vi "Generate Dep Links.vi"(8 "error in":errorcluster, 9 "Dependency Names":string[](array[string]), 10 "Name":string, 11 "Create Unowned Container?":bool) -> (0 "error out":errorcluster, 3 "DGML Link Strings":string[](array[string]))   [LabVIEW 2018, in "DGML creation.lvlib"]
uses:
  DGML creation.lvlib
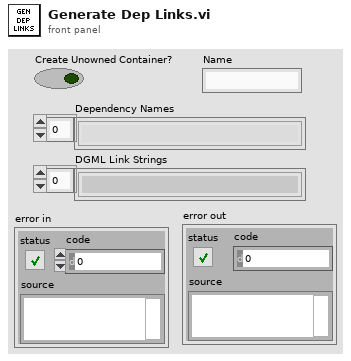
[diagram p1: front panel]
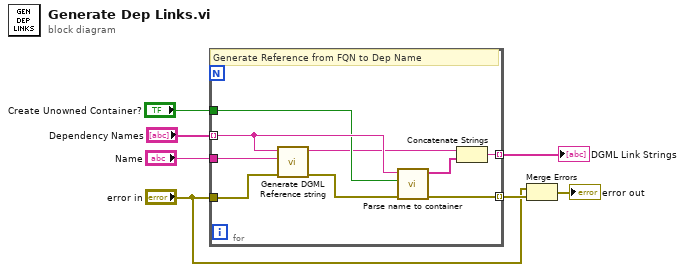
[diagram p0: block diagram]
diagram:
  n1 = for {
    tunnel: "Dependency Names" -> [w14] mode=indexing
    tunnel: "Name" -> [w16]
    tunnel: [w15] -> w5 mode=indexing
    tunnel: "Create Unowned Container?" -> [w12]
    tunnel: "error in" -> [w11]
    tunnel: [w8] -> w3 mode=indexing
    # "Generate Reference from FQN to Dep Name"
    n2 = call "Generate DGML Reference string.vi"("error in (no error)"=w11, "Name"=w16, "String in"=w14) -> ("error out"=w9:errorcluster, "String out"=w10:string)  [unwired: 7 in]
    n3 = call "Parse name to container.vi"("error in"=w9, "Create Unowned Container?"=w12, "Fully Qualified Name"=w14) -> ("error out"=w8:errorcluster, "Container DGML Strings"=w13:string[])  [unwired: 7 in]
    n4 = Concatenate Strings(w10, w13) -> (w15:string)
  }
  "DGML Link Strings" <- w5
  n5 = Merge Errors("error in", w3) -> (→"error out":errorcluster)
